vi "Shutdown App.vi"(8 "error in":errorcluster, 11 "Peer Review in":refnum<class "Peer Review.lvclass">) -> (0 "error out":errorcluster, 3 "Peer Review out":refnum<class "Peer Review.lvclass">)   [LabVIEW 2020, in "Peer Review.lvclass"]
uses:
  Peer Review.lvclass
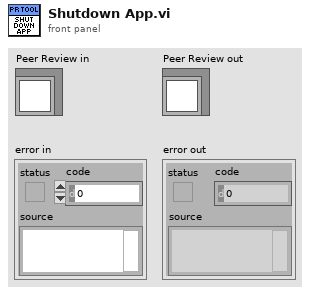
[diagram p1: front panel]
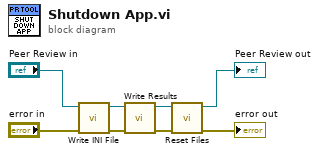
[diagram p0: block diagram]
diagram:
  n1 = call "Write INI File.vi"("error in"="error in", "Peer Review in"="Peer Review in") -> ("error out"=w7:errorcluster, "Peer Review out"=w5:refnum<class "Peer Review.lvclass">)  [unwired: 8 in]
  n2 = call "Write Results.vi"("error in"=w7, "Peer Review in"=w5) -> ("error out"=w4:errorcluster, "Peer Review out"=w2:refnum<class "Peer Review.lvclass">)  [unwired: 8 in]
  n3 = call "Reset Files.vi"("error in"=w4, "Peer Review in"=w2) -> ("error out"=→"error out":errorcluster, "Peer Review out"=→"Peer Review out":refnum<class "Peer Review.lvclass">)  [unwired: 8 in]
